vi "Cleanup.vi"(8 "error in (no error)":errorcluster, 11 "FTP in":refnum<class "FTP.lvclass">) -> (0 "error out":errorcluster, 3 "FTP out":refnum<class "FTP.lvclass">)   [LabVIEW 2017, in "FTP_UpgradeCSMF.lvlib" / "FTP.lvclass"]
uses:
  FTP.lvclass
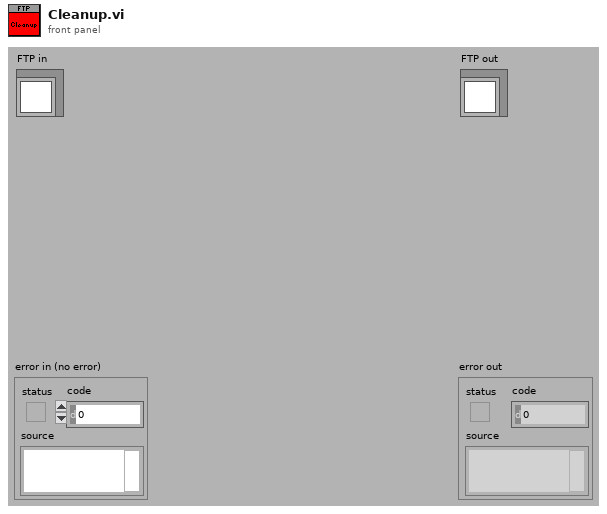
[diagram p1: front panel]
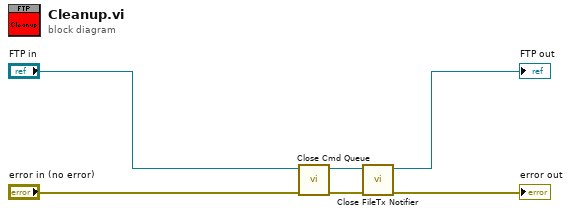
[diagram p0: block diagram]
diagram:
  n1 = call "Close Cmd Queue.vi"("error in (no error)"="error in (no error)", "FTP in"="FTP in") -> ("error out"=w6:errorcluster, "FTP out"=w5:refnum<class "FTP.lvclass">)  [unwired: 8 in]
  n2 = call "Close FileTx Notifier.vi"("error in (no error)"=w6, "FTP in"=w5) -> ("error out"=→"error out":errorcluster, "FTP out"=→"FTP out":refnum<class "FTP.lvclass">)  [unwired: 8 in]
